vi "LKIF_GetCalcData.vi"(8 "error in (no error)":errorcluster {"code" format="%x"}) -> (0 "error out":errorcluster {"code" format="%x"}, 2 "CalcData2":T1 {"LKIF_FLOATRESULT" items=["VALID", "RANGEOVER_P", "RANGEOVER_N", "WAITING"]}, 3 "CalcData1":T1 {"LKIF_FLOATRESULT" items=["VALID", "RANGEOVER_P", "RANGEOVER_N", "WAITING"]})   [LabVIEW 8.6, in "Keyence LK-G3000.lvlib"]
uses:
  Keyence LK-G3000.lvlib
  enums/LKIF_FLOATRESULT.ctl
  clusters/LKIF_FLOATVALUE.ctl
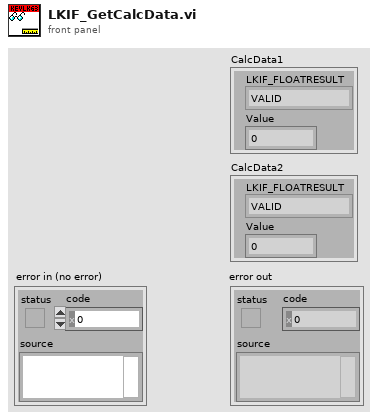
[diagram p1: front panel]
types:
  T1 = typedef "Keyence LK-G3000.lvlib/LKIF_FLOATVALUE.ctl" = cluster{"LKIF_FLOATRESULT":T2, "Value":sgl}
  T2 = typedef "Keyence LK-G3000.lvlib/LKIF_FLOATRESULT.ctl" = i32
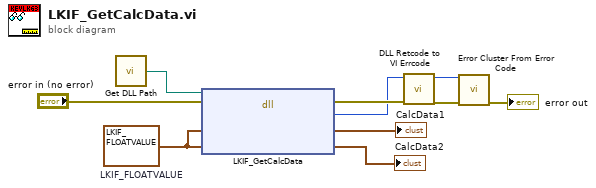
[diagram p0: block diagram]
diagram:
  w3 = T1 ?  # LKIF_FLOATVALUE
  n1 = call "Get DLL Path.vi"() -> ("DLL Path"=w4:path)  [unwired: 1 in]
  n2 = dll-call lib="C:/Program Files/National Instruments/LabVIEW 2011/instr.lib/Keyence LK-G3000/LkIF.dll" fn="LKIF_GetCalcData"(path in=w4, error in="error in (no error)", "CalcData1"=w3, "CalcData2"=w3) -> (error out=w7:errorcluster, "RC"=w6:i32, "CalcData1"=→"CalcData1":T1, "CalcData2"=→"CalcData2":T1)  [unwired: 1 in, 1 out]
  n3 = call "DLL Retcode to VI Errcode.vi"("error in (no error)"=w7, "DLL Retcode"=w6) -> ("error out"=w10:errorcluster, "VI Errcode"=w9:i32)  [unwired: 8 in]
  n4 = call <vilib>:"Error Cluster From Error Code.vi"("error in (no error)"=w10, "error code (0)"=w9) -> ("error out"=→"error out":errorcluster)  [unwired: 7 in]
